vi "FITS - Format FITS Keyword v2 .vi"(0 "Keyword":string="BITPIX", 1 "Value":string="16", 2 "Comment":string="BITS PER PIXEL") -> (3 "Formatted fits entry":string="BITPIX  =                   16 / BITS PER PIXEL                                 ", 5 "Length of line":i16=80)   [LabVIEW 2014]
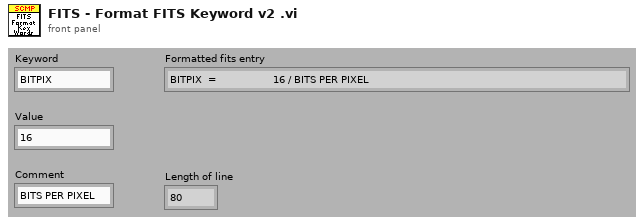
[diagram p1: front panel]
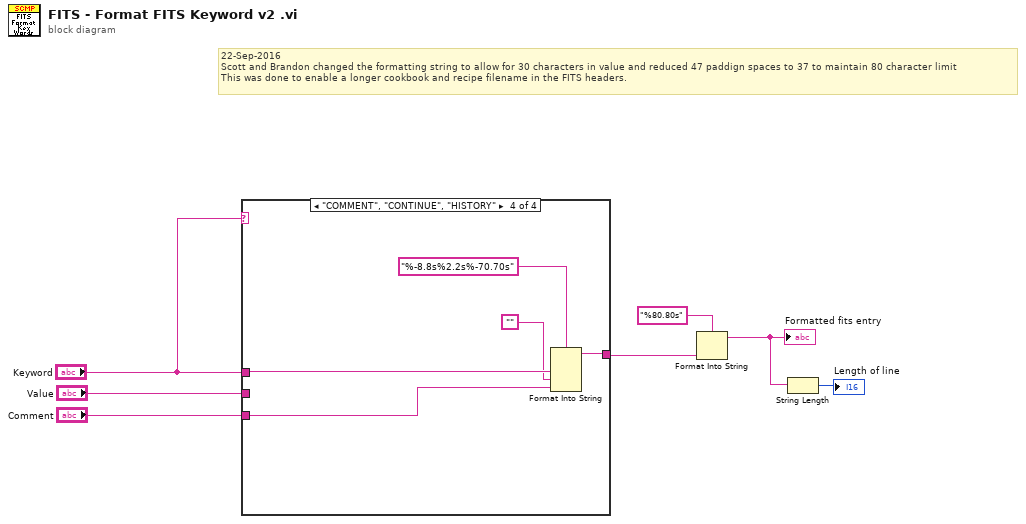
[diagram p0: block diagram]
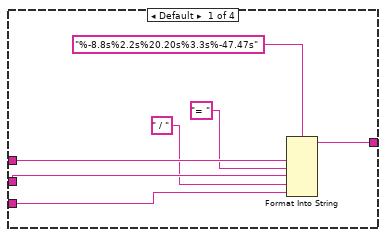
[diagram p2: hidden frame]
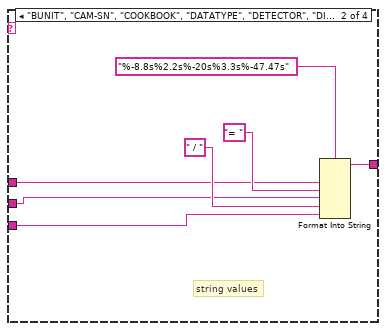
[diagram p3: hidden frame]
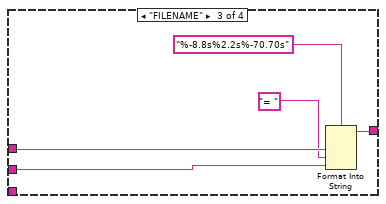
[diagram p4: hidden frame]
diagram:
  # "22-Sep-2016\nScott and Brandon changed the formatting string to allow for 30 characters in value and reduced 47 paddign spaces to 37 to maintain 80 character limit\nThis was done to enable a longer cookbook and recipe filename in the FITS headers."
  n1 = case shown="\"COMMENT\", \"CONTINUE\", \"HISTORY\"" "Keyword" {
    tunnel: "Value" -> [w13 w17 w24 _]
    tunnel: "Keyword" -> [w12 w18 w25 w30]
    tunnel: "Comment" -> [w9 w16 _ w27]
    tunnel: [w8 w15 w22 w31] -> w3
    frame Default {
      n2 = Format Into String(format string="%-8.8s%2.2s%20.20s%3.3s%-47.47s", w12, "= ", w13, " / ", w9) -> (resulting string=w8:string)  [unwired: 2 in, 1 out]
    }
    frame "BUNIT", "CAM-SN", "COOKBOOK", "DATATYPE", "DETECTOR", "DIFFUSER", "FILTER", "FLC-1", "FLC-2", "FW-CALIB", "INSTRUME", "LOCATION", "OBSERVER", "OBS_PROG", "ORIGIN", "TELESCOP", "TIMESYS" {
      # "string values"
      n3 = Format Into String(format string="%-8.8s%2.2s%-20s%3.3s%-47.47s", w18, "= ", w17, " / ", w16) -> (resulting string=w15:string)  [unwired: 2 in, 1 out]
    }
    frame "FILENAME" {
      n4 = Format Into String(format string="%-8.8s%2.2s%-70.70s", w25, "= ", w24) -> (resulting string=w22:string)  [unwired: 2 in, 1 out]
    }
    frame "COMMENT", "CONTINUE", "HISTORY" {
      n5 = Format Into String(format string="%-8.8s%2.2s%-70.70s", w30, "", w27) -> (resulting string=w31:string)  [unwired: 2 in, 1 out]
    }
  }
  n6 = Format Into String(format string="%80.80s" ("initial string"), w3) -> (resulting string=w2:string)  [unwired: 2 in, 1 out]
  "Formatted fits entry" <- w2
  n7 = String Length(string=w2) -> (length=→"Length of line":i32)
